vi "MI.Get Chamber Pressure.vi"(8 "error in (no error)":errorcluster, 11 "TCP Network Connection in":refnum<k5>) -> (0 "error out":errorcluster, 2 "Chamber Pressure (mTorr)":dbl, 3 "TCP Network Connection out":refnum<k5>)   [LabVIEW 2016, in "instrument.Cryostation.lvclass"]
uses:
  instrument.Cryostation.lvclass
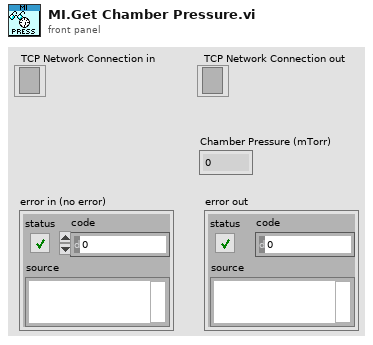
[diagram p1: front panel]
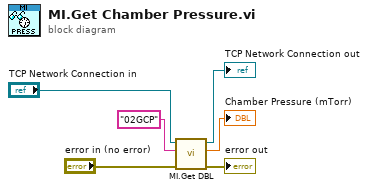
[diagram p0: block diagram]
diagram:
  n1 = call "MI.Get DBL.vi"("error in (no error)"="error in (no error)", "String"="02GCP", "TCP Network Connection in"="TCP Network Connection in") -> ("error out"=→"error out":errorcluster, "Numeric"=→"Chamber Pressure (mTorr)":dbl, "TCP Network Connection out"=→"TCP Network Connection out":refnum<k5>)  [unwired: 6 in]
